vi "2DTrainedRegression.vi"(8 "error in":errorcluster, 11 "Parameters":T6={"Plot"=refnum, "Data"={"Split"={"X Train"=[], "X Test"=[], "Y Train"=[], "Y Test"=[]}, "Predict"=[]}, "Display"={"Choice"=enum."All", "Indexe"={"X"=0, "Y"=1}}, "Point Property"={"Train Style"=enum."Full circle", "Test OK Style"=enum."Full square", "Label Color"=[8978528, 4367871, 16716800], "Test NO OK"={"Style"=enum."Cross", "Color"=16711680}}, "Tolerance's threshold"=0.0}) -> (0 "error out":errorcluster)   [LabVIEW 2020]
uses:
  _Controls/Datas.ctl
  _Controls/PointPropertyMultipleLabel.ctl
  _Controls/Style.ctl
  _Controls/2DData.ctl
panel:
  in  "Local":T5={"Parameters"={"Plot"=refnum, "Data"={"Split"={"X Train"=[], "X Test"=[], "Y Train"=[], "Y Test"=[]}, "Predict"=[]}, "Display"={"Choice"=enum."All", "Indexe"={"X"=0, "Y"=1}}, "Point Property"={"Train Style"=enum."Full circle", "Test OK Style"=enum."Full square", "Label Color"=[8978528, 4367871, 16716800], "Test NO OK"={"Style"=enum."Cross", "Color"=16711680}}, "Tolerance's threshold"=0.0}, "2D Array"=[], "Point ID"=[], "GoodPredict"=0, "Rating 2D Array"=[]}
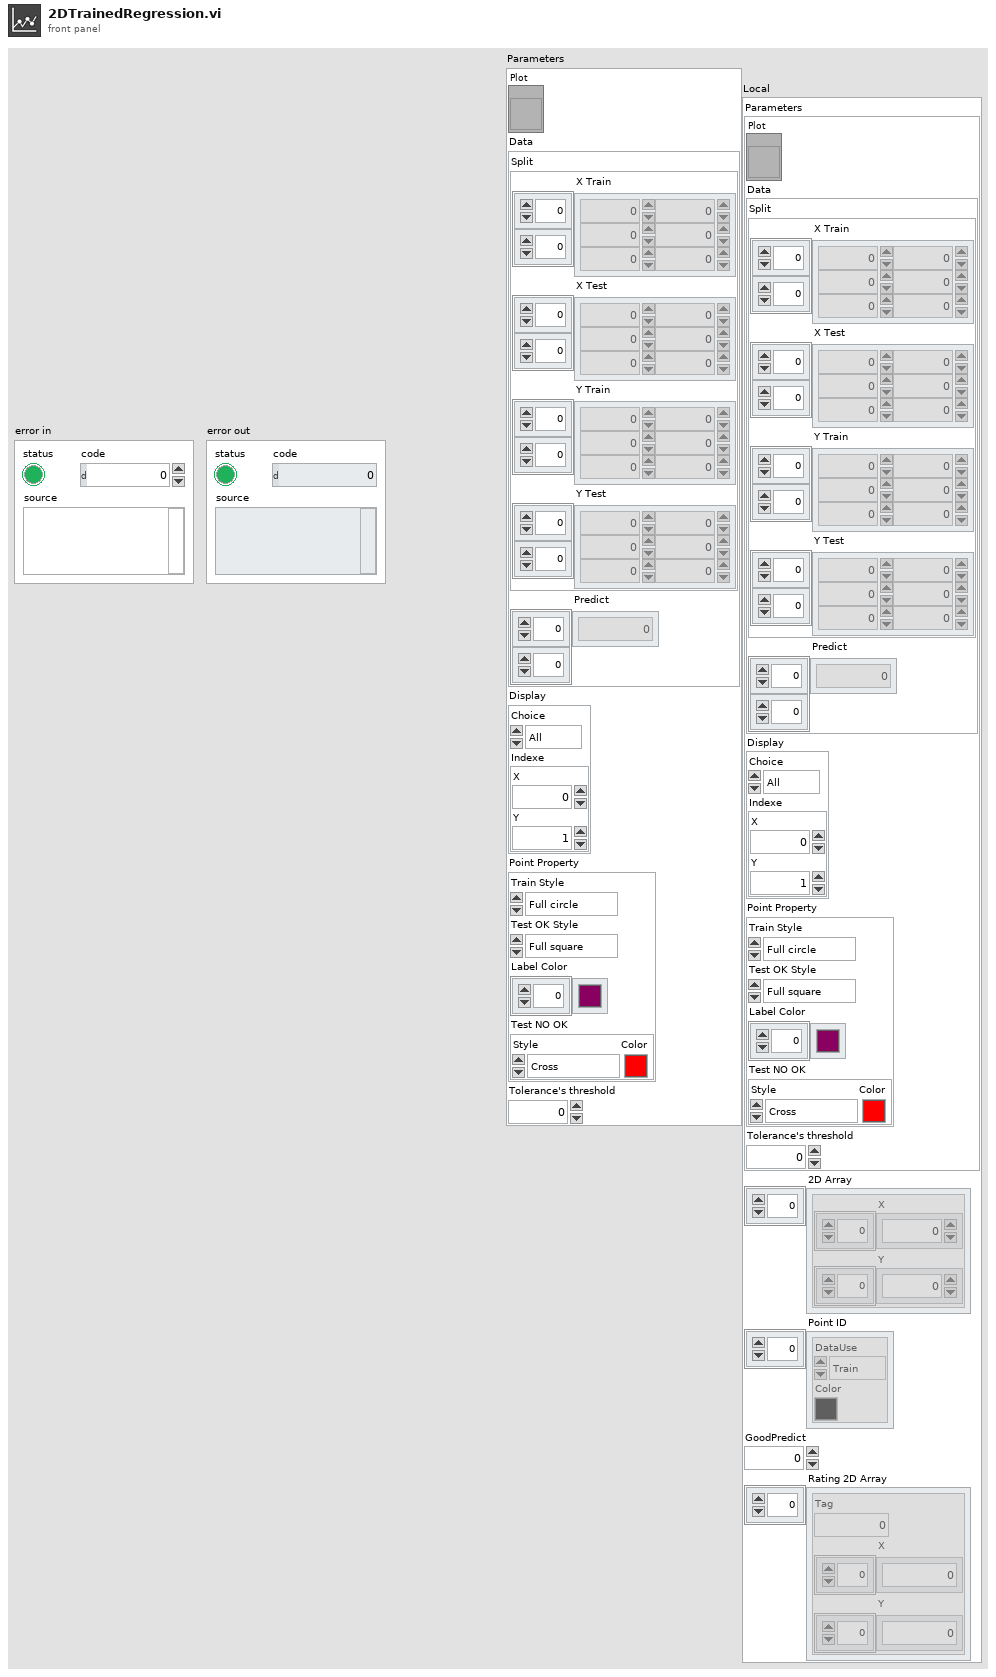
[diagram p1: front panel]
types:
  T1 = typedef "Datas.ctl" = cluster{"Split":cluster{"X Train":dbl[][], "X Test":dbl[][], "Y Train":dbl[][], "Y Test":dbl[][]}, "Predict":dbl[][]}
  T2 = typedef "PointPropertyMultipleLabel.ctl" = cluster{"Train Style":T3, "Test OK Style":T3, "Label Color":u32[], "Test NO OK":cluster{"Style":T3, "Color":u32}}
  T3 = typedef "Style.ctl" = enum16{"Empty circle", "Full circle", "Empty square", "Full square", "Cross"}
  T4 = typedef "2DData.ctl" = cluster{"Tag":i32, "X":dbl[], "Y":dbl[]}
  T5 = cluster{"Parameters":cluster{"Plot":refnum<vi>, "Data":T1, "Display":cluster{"Choice":enum16{"All", "Train", "Test"}, "Indexe":cluster{"X":i32, "Y":i32}}, "Point Property":T2, "Tolerance's threshold":dbl}, "2D Array":cluster{"X":dbl[], "Y":dbl[]}[], "Point ID":cluster{"DataUse":enum16{"Dataset", "Train", "Test"}, "Color":u32}[], "GoodPredict":i32, "Rating 2D Array":T4[]}
  T6 = cluster{"Plot":refnum<vi>, "Data":T1, "Display":cluster{"Choice":enum16{"All", "Train", "Test"}, "Indexe":cluster{"X":i32, "Y":i32}}, "Point Property":T2, "Tolerance's threshold":dbl}
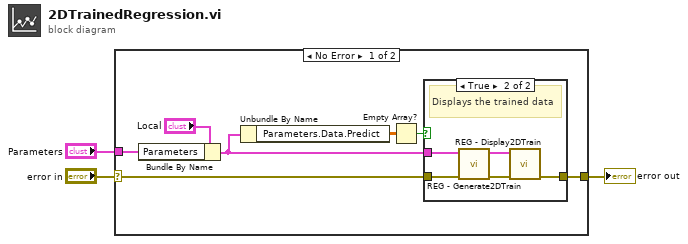
[diagram p0: block diagram]
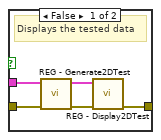
[diagram p2: hidden frame]
diagram:
  n1 = case shown="No Error" "error in" {
    selector: "error in" -> [w6 w21]
    tunnel: [w5 w21] -> w2
    tunnel: "Parameters" -> [w4 _]
    frame No Error {
      n2 = Bundle By Name(cluster="Local", "Parameters"=w4) -> (w10:T5)
      n3 = Unbundle By Name(w10) -> ("Parameters.Data.Predict"=w9:dbl[][])
      n4 = Empty Array?(array=w9) -> (empty?=w8:bool)
      n5 = case shown="True" w8 {
        tunnel: w6 -> [w14 w19]
        tunnel: [w12 w16] -> w5
        tunnel: w10 -> [w15 w20]
        frame False {
          # "Displays the tested data"
          n6 = call "REG - Generate2DTest.vi"("error in (no error)"=w14, "Local"=w15) -> ("error out"=w13:errorcluster, "Local Out"=w11:T5)  [unwired: 8 in]
          n7 = call "REG - Display2DTest.vi"("error in"=w13, "Local"=w11) -> ("error out"=w12:errorcluster)  [unwired: 8 in, 1 out]
        }
        frame True {
          # "Displays the trained data"
          n8 = call "REG - Generate2DTrain.vi"("error in"=w19, "Local"=w20) -> ("error out"=w17:errorcluster, "Local_Out"=w18:T5)  [unwired: 8 in]
          n9 = call "REG - Display2DTrain.vi"("error in"=w17, "Local"=w18) -> ("error out"=w16:errorcluster)  [unwired: 8 in, 1 out]
        }
      }
    }
    frame Error {
    }
  }
  "error out" <- w2
